vi "ProgrammaticBuildBuild.vi"() -> ()   [LabVIEW 2021]
uses:
  <vilib>/AppBuilder/AB_API_Simple/Build (path).vi
  <vilib>/AppBuilder/AB_API_Simple/NI_App_Builder_API.lvlib
panel:
  out "error out":errorcluster
  out "Generated files":path[](array[path])
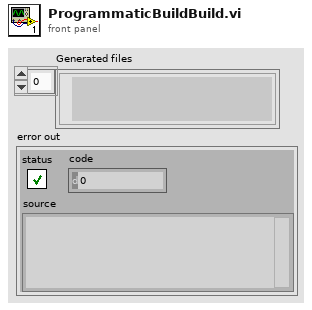
[diagram p1: front panel]
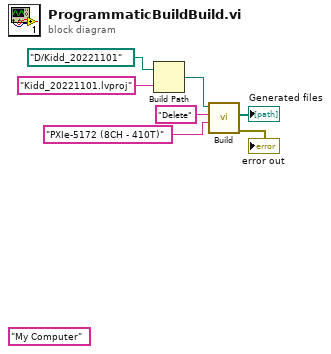
[diagram p0: block diagram]
diagram:
  (unwired) "My Computer" ("Name of target (My Computer)")
  n1 = Build Path(base path=path "D:/Kidd_20221101", name or relative path="Kidd_20221101.lvproj") -> (appended path=w5:path)
  n2 = call-poly <vilib>:"Build.vi"("Name of target (My Computer)"="PXIe-5172 (8CH - 410T)", "Name of build specification (if empty: build all)"="Delete", "Path to project"=w5) -> ("error out"=→"error out":errorcluster, "Generated files"=→"Generated files":path[])  [unwired: 7 in]
